vi "Micronix Approach Main - Digital Pulse.vi"() -> ()   [LabVIEW 2021]
panel:
  in  "Polarity":bool caption="pos      neg"
  in  "Controller #":string
  in  "Pulse In":tag
  in  "rate":dbl=1000.0
  in  "Reset":bool
  in  "Stop":bool
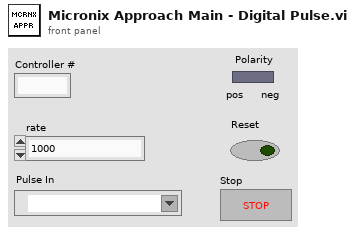
[diagram p1: front panel]
types:
  T1 = cluster{"P type":u16, "VISA resource name out":refnum<visa-resource-name>, " Terminator":string, "Timeout":i32}
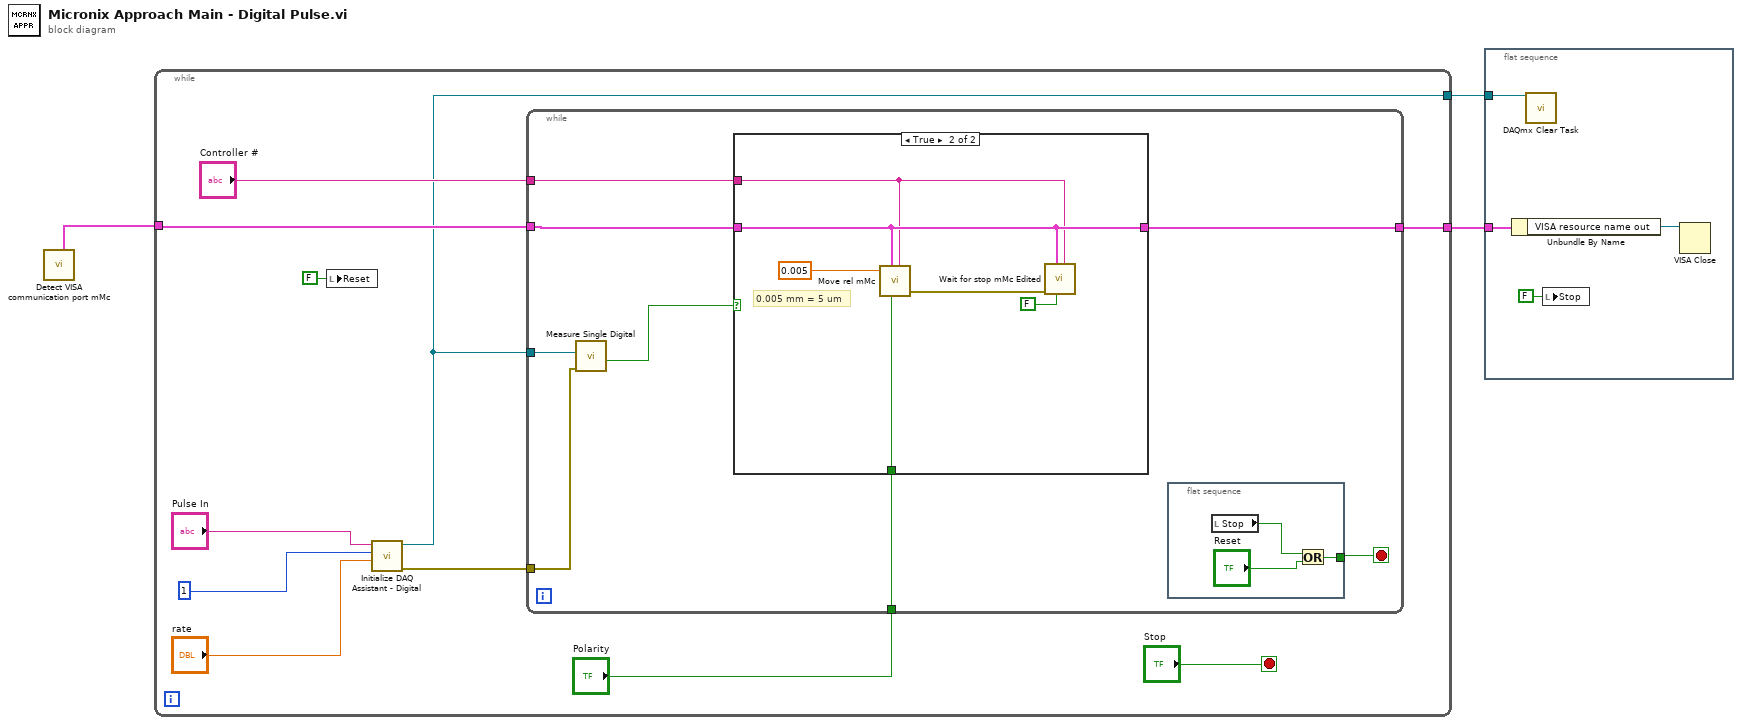
[diagram p0: block diagram]
diagram:
  n1 = call "Detect VISA communication port mMc.vi"() -> ("Port"=w3:T1)  [unwired: 6 in, 3 out]
  n2 = while {
    tunnel: w3 -> [w13]
    tunnel: [w5] -> w2
    tunnel: [w10] -> w1
    stop <- "Stop" stop-if-true
    n3 = local write "Reset"(FALSE ("Reset")) -> ()
    n4 = call "Initialize DAQ Assistant - Digital.vi"("rate"="rate", "number of samples"=1, "physical channels"="Pulse In") -> ("error out"=w4:errorcluster, "task out"=w5:refnum<k21>)  [unwired: 7 in]
    n5 = while {
      tunnel: w13 -> [w22]
      tunnel: [w20] -> w10
      tunnel: "Controller #" -> [w19]
      tunnel: "Polarity" -> [w18]
      tunnel: w5 -> [w17]
      tunnel: w4 -> [w16]
      stop <- w21 stop-if-true
      n6 = call "Measure Single Digital.vi"("error in"=w16, "task/channels in"=w17) -> ("data"=w15:bool)  [unwired: 7 in, 2 out]
      n7 = case shown="True" w15 {
        tunnel: w22 -> [w26 w29]
        tunnel: [w26 w29] -> w20
        tunnel: w19 -> [_ w27]
        tunnel: w18 -> [_ w28]
        frame False {
        }
        frame True {
          # "0.005 mm = 5 um"
          n8 = call "Move rel mMc.vi"("position incr"=0.005, "Port"=w29, "rev dir?"=w28, "Controller #"=w27) -> ("error out"=w32:errorcluster)  [unwired: 5 in]
          n9 = call "Wait for stop mMc Edited.vi"("Controller #"=w27, "wait for in pos"=FALSE, "Port"=w29, "error in (no error)"=w32) -> ()  [unwired: 7 in, 1 out]
        }
      }
      n10 = flat-sequence {
        tunnel: [w25] -> w21
        frame #0 {
          n11 = local read "Stop"() -> (w23:bool)
          n12 = Or(x=w23, y="Reset") -> (x .or. y?=w25:bool)
        }
      }
    }
  }
  n13 = flat-sequence {
    tunnel: w2 -> [w36]
    tunnel: w1 -> [w34]
    frame #0 {
      n14 = Unbundle By Name(w34) -> ("VISA resource name out"=w35:refnum<visa-resource-name>)
      n15 = call <vilib>:"DAQmx Clear Task.vi"("task in"=w36) -> ()  [unwired: 14 in, 1 out]
      n16 = local write "Stop"(FALSE ("Stop")) -> ()
      n17 = VISA Close(VISA resource name=w35) -> ()  [unwired: 1 in, 1 out]
    }
  }
